vi "PH_Sound.Ice Hockey 3.vi"() -> (0 "Ice Hockey 3":cluster{"Tone":dbl, "Beats":i32}[](array[cluster]))   [LabVIEW 2014, in "PH_Sound.lvlib"]
doc: "\"Alle Vögel sind schon da, ...\""
uses:
  PH_Sound.lvlib
  PH_Sound.3Oktaves.ctl
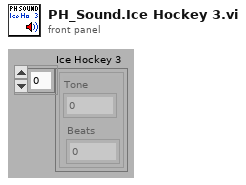
[diagram p1: front panel]
types:
  T1 = typedef "PH_Sound.lvlib/PH_Sound.3Oktaves.ctl" = dbl
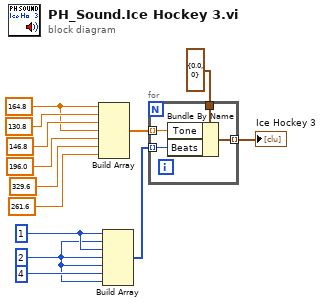
[diagram p0: block diagram]
diagram:
  w5 = T1 261.6 items=["c"=130.8, "cis"=138.6, "d"=146.8, "es"=155.6, "e"=164.8, "f"=174.6, "fis"=185.0, "g"=196.0, "as"=207.6, "a"=220.0, "b"=233.1, "h"=246.9, "c'"=261.6, "cis'"=277.2, "d'"=293.7, "es'"=311.1, "e'"=329.6, "f'"=349.2, "fis'"=370.0, "g'"=392.0, "as'"=415.3, "a'"=440.0, "b'"=466.2, "h'"=493.9, "c''"=523.3, "cis''"=554.4, "d''"=587.3, "es''"=622.3, "e''"=659.3, "f''"=689.5, "fis''"=740.0, "g''"=784.0, "as''"=830.6, "a''"=880.0, "b''"=932.3, "h''"=987.8, "c'''"=1047.0] ("3 Octaves")
  w6 = T1 329.6 items=["c"=130.8, "cis"=138.6, "d"=146.8, "es"=155.6, "e"=164.8, "f"=174.6, "fis"=185.0, "g"=196.0, "as"=207.6, "a"=220.0, "b"=233.1, "h"=246.9, "c'"=261.6, "cis'"=277.2, "d'"=293.7, "es'"=311.1, "e'"=329.6, "f'"=349.2, "fis'"=370.0, "g'"=392.0, "as'"=415.3, "a'"=440.0, "b'"=466.2, "h'"=493.9, "c''"=523.3, "cis''"=554.4, "d''"=587.3, "es''"=622.3, "e''"=659.3, "f''"=689.5, "fis''"=740.0, "g''"=784.0, "as''"=830.6, "a''"=880.0, "b''"=932.3, "h''"=987.8, "c'''"=1047.0] ("3 Octaves")
  w2 = 2 ("element")
  w4 = 1 ("y")
  w7 = T1 196.0 items=["c"=130.8, "cis"=138.6, "d"=146.8, "es"=155.6, "e"=164.8, "f"=174.6, "fis"=185.0, "g"=196.0, "as"=207.6, "a"=220.0, "b"=233.1, "h"=246.9, "c'"=261.6, "cis'"=277.2, "d'"=293.7, "es'"=311.1, "e'"=329.6, "f'"=349.2, "fis'"=370.0, "g'"=392.0, "as'"=415.3, "a'"=440.0, "b'"=466.2, "h'"=493.9, "c''"=523.3, "cis''"=554.4, "d''"=587.3, "es''"=622.3, "e''"=659.3, "f''"=689.5, "fis''"=740.0, "g''"=784.0, "as''"=830.6, "a''"=880.0, "b''"=932.3, "h''"=987.8, "c'''"=1047.0] ("3 Octaves")
  w10 = T1 146.8 items=["c"=130.8, "cis"=138.6, "d"=146.8, "es"=155.6, "e"=164.8, "f"=174.6, "fis"=185.0, "g"=196.0, "as"=207.6, "a"=220.0, "b"=233.1, "h"=246.9, "c'"=261.6, "cis'"=277.2, "d'"=293.7, "es'"=311.1, "e'"=329.6, "f'"=349.2, "fis'"=370.0, "g'"=392.0, "as'"=415.3, "a'"=440.0, "b'"=466.2, "h'"=493.9, "c''"=523.3, "cis''"=554.4, "d''"=587.3, "es''"=622.3, "e''"=659.3, "f''"=689.5, "fis''"=740.0, "g''"=784.0, "as''"=830.6, "a''"=880.0, "b''"=932.3, "h''"=987.8, "c'''"=1047.0] ("3 Octaves")
  w13 = T1 130.8 items=["c"=130.8, "cis"=138.6, "d"=146.8, "es"=155.6, "e"=164.8, "f"=174.6, "fis"=185.0, "g"=196.0, "as"=207.6, "a"=220.0, "b"=233.1, "h"=246.9, "c'"=261.6, "cis'"=277.2, "d'"=293.7, "es'"=311.1, "e'"=329.6, "f'"=349.2, "fis'"=370.0, "g'"=392.0, "as'"=415.3, "a'"=440.0, "b'"=466.2, "h'"=493.9, "c''"=523.3, "cis''"=554.4, "d''"=587.3, "es''"=622.3, "e''"=659.3, "f''"=689.5, "fis''"=740.0, "g''"=784.0, "as''"=830.6, "a''"=880.0, "b''"=932.3, "h''"=987.8, "c'''"=1047.0] ("3 Octaves")
  w8 = T1 164.8 items=["c"=130.8, "cis"=138.6, "d"=146.8, "es"=155.6, "e"=164.8, "f"=174.6, "fis"=185.0, "g"=196.0, "as"=207.6, "a"=220.0, "b"=233.1, "h"=246.9, "c'"=261.6, "cis'"=277.2, "d'"=293.7, "es'"=311.1, "e'"=329.6, "f'"=349.2, "fis'"=370.0, "g'"=392.0, "as'"=415.3, "a'"=440.0, "b'"=466.2, "h'"=493.9, "c''"=523.3, "cis''"=554.4, "d''"=587.3, "es''"=622.3, "e''"=659.3, "f''"=689.5, "fis''"=740.0, "g''"=784.0, "as''"=830.6, "a''"=880.0, "b''"=932.3, "h''"=987.8, "c'''"=1047.0] ("3 Octaves")
  n1 = Build Array(w8, w13, w10, w8, w7, w6, w5) -> (w12:T1[])
  n2 = Build Array(w4, w2, w4, w2, w2, 4 ("element"), w2) -> (w1:i32[])
  n3 = for {
    tunnel: w12 -> [w16] mode=indexing
    tunnel: cluster{"Tone":dbl, "Beats":i32} {"Tone"=0.0, "Beats"=0} ("Note") -> [w17]
    tunnel: [w15] -> w11 mode=indexing
    tunnel: w1 -> [w14] mode=indexing
    n4 = Bundle By Name(cluster=w17, "Tone"=w16, "Beats"=w14) -> (w15:cluster{"Tone":dbl, "Beats":i32})
  }
  "Ice Hockey 3" <- w11
